vi "Debug Spy.vi"(8 "error in (no error)":errorcluster, 9 "Message Data":variant, 10 "Message":string, 11 "Process in":refnum<class "Process.lvclass">) -> (0 "error out":errorcluster, 1 "Message Data dup":variant, 2 "Message dup":string, 3 "Process out":refnum<class "Process.lvclass">)   [LabVIEW 2020, in "Process.lvclass"]
uses:
  Process.lvclass
  Logging/Logging.lvclass
  C:/Users/anton/Documents/GitHub/Triarc-Framework/source/Framework/Base/Base.lvclass
  C:/Users/anton/Documents/GitHub/Triarc-Framework/source/Framework/Process/Process.lvclass
  C:/Users/anton/Documents/GitHub/Triarc-Framework/source/Framework/Error Handler Interface/Error Handler Interface.lvclass
  C:/Users/anton/Documents/GitHub/Triarc-Framework/source/Framework/Logging/Logging.lvclass
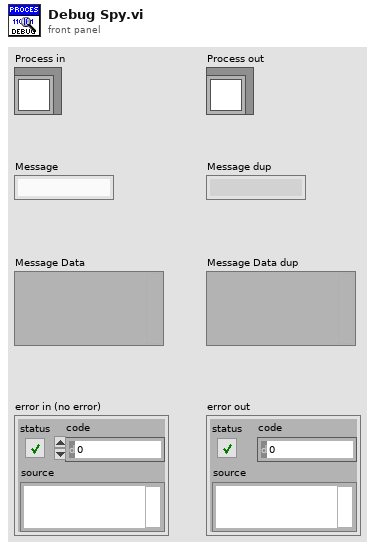
[diagram p1: front panel]
types:
  T1 = cluster{"Action":string, "Call Chain":string, "Process":string, "Message":string, "Message Data":variant, "Time":u32}
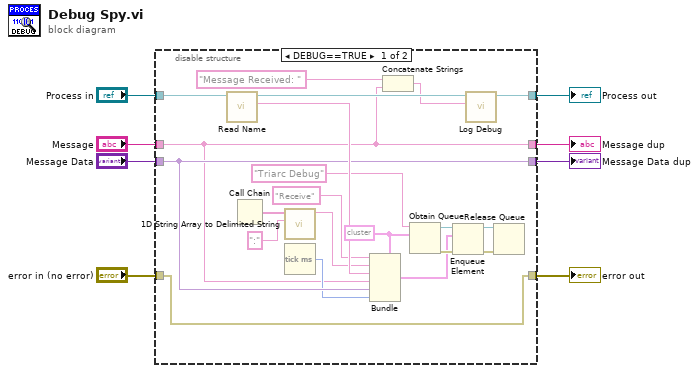
[diagram p0: block diagram]
diagram:
  n1 = disable-structure shown="DEBUG==TRUE" {
    disable-tunnel: "Message" -> [w9 w33]
    disable-tunnel: "Message Data" -> [w16 w32]
    disable-tunnel: [w16 w32] -> w3
    disable-tunnel: [w9 w33] -> w4
    disable-tunnel: [w12 w31] -> w5
    disable-tunnel: "Process in" -> [w14 w31]
    disable-tunnel: [w17 w30] -> w6
    disable-tunnel: "error in (no error)" -> [w17 w30]
    frame condition #0 {
      w24 = T1 {"Action"="", "Call Chain"="", "Process"="", "Message"="", "Message Data"=variant, "Time"=0} ("output cluster")
      n2 = call-dynamic "Read Name.vi"("Process In"=w14) -> ("Qualified Name"=w29:string, "Process Out"=w15:refnum<class "Process.lvclass">)  [unwired: 7 in, 2 out]
      n3 = Call Chain() -> (call chain=w28:string[])
      n4 = call <vilib>:"1D String Array to Delimited String.vi"("delimiter"=":", "string array"=w28) -> ("delimited string"=w26:string)  [unwired: 9 in]
      n5 = Tick Count (ms)() -> (millisecond timer value=w13:u32)
      n6 = Bundle(cluster=w24, "Action"="Receive", "Call Chain"=w26, "Process"=w29, "Message"=w9, "Message Data"=w16, "Time"=w13) -> (w21:T1)
      n7 = Concatenate Strings("Message Received: " ("name (unnamed)"), w9) -> (w10:string)
      n8 = Obtain Queue(name (unnamed)="Triarc Debug", element data type=w24) -> (queue out=w23:refnum<queue>, error out=w22:errorcluster)  [unwired: 3 in, 1 out]
      n9 = Enqueue Element(queue=w23, element=w21, error in (no error)=w22) -> (queue out=w20:refnum<queue>, error out=w19:errorcluster)  [unwired: 1 in, 1 out]
      n10 = call "Log Debug.vi"("Message"=w10, "Logging In"=w15) -> ("Logging Out"=w12:refnum<class "Process.lvclass">)  [unwired: 8 in, 1 out]
      n11 = Release Queue(queue=w20, error in (no error)=w19) -> ()  [unwired: 1 in, 3 out]
    }
    frame condition #1 (active) {
    }
  }
  "error out" <- w6
  "Process out" <- w5
  "Message dup" <- w4
  "Message Data dup" <- w3
